vi "CreateDicomPath.vi"(8 "error in (no error)":errorcluster, 10 "Measurement ID":string, 11 "patientID":string) -> (0 "error out":errorcluster, 2 "Path":path, 3 "String":string)   [LabVIEW 2013, in "main.lvlib"]
uses:
  main.lvlib
  Globals/DataPathGlobalVariable.vi
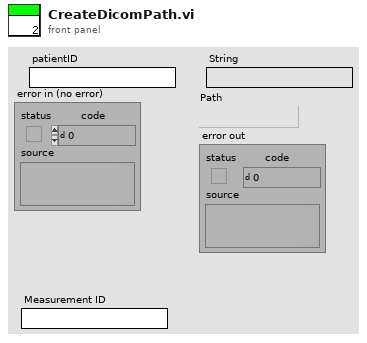
[diagram p1: front panel]
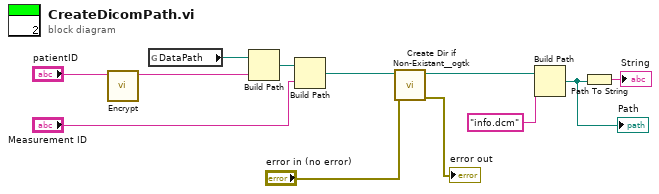
[diagram p0: block diagram]
diagram:
  n1 = call "Encrypt.vi"("Input"="patientID") -> ("Output"=w7:string)  [unwired: 10 in]
  n2 = global read "DataPathGlobalVariable.vi" "DataPath"() -> (w4:path)
  n3 = Build Path(base path=w4, name or relative path=w7) -> (appended path=w5:path)
  n4 = Build Path(base path=w5, name or relative path="Measurement ID") -> (appended path=w8:path)
  n5 = call <userlib>:"Create Dir if Non-Existant__ogtk.vi"("error in (no error)"="error in (no error)", "Directory Path"=w8) -> ("error out"=→"error out":errorcluster, "dup Directory Path"=w9:path)  [unwired: 7 in, 1 out]
  n6 = Build Path(base path=w9, name or relative path="info.dcm") -> (appended path=w11:path)
  "Path" <- w11
  n7 = Path To String(path=w11) -> (string=→"String":string)
